vi "Measure Delay.vi"(0 "Oscilloscope in":refnum<class "Oscilloscope.lvclass">, 1 "From Slope Edge":T2, 5 "From Channel":T3, 7 "To Channel":T3, 9 "No. Reads":i32, 11 "error in (no error)":errorcluster, 12 "To Slope Edge":T2) -> (4 "Oscilloscope out":refnum<class "Oscilloscope.lvclass">, 6 "Statistics":T1, 15 "error out":errorcluster)   [LabVIEW 2018, in "Oscilloscope.lvlib" / "Oscilloscope.lvclass"]
doc: "This Override measure the signal time gap between From Channel's Slope Edge to To Channel's Slope Edge."
uses:
  Oscilloscope.lvclass
  Custom Controls/Analog Channels.ctl
  Custom Controls/Slope Edge.ctl
  Oscilloscope.lvlib
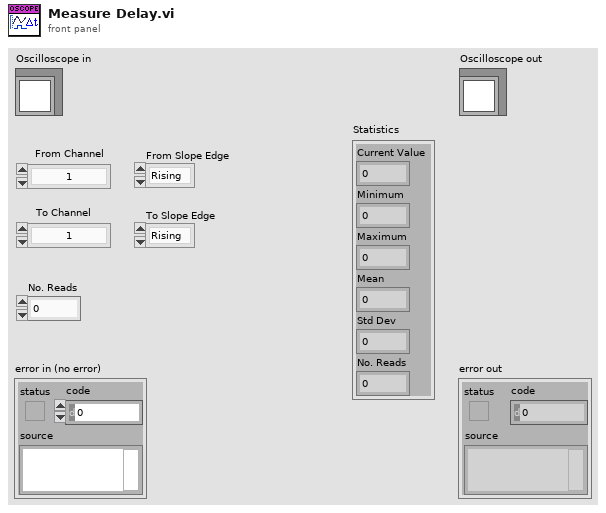
[diagram p1: front panel]
types:
  T1 = cluster{"Current Value":dbl, "Minimum":dbl, "Maximum":dbl, "Mean":dbl, "Std Dev":dbl, "No. Reads":dbl}
  T2 = typedef "Oscilloscope.lvlib/Slope Edge.ctl" = enum16{"Rising", "Falling"}
  T3 = typedef "Oscilloscope.lvlib/Analog Channels.ctl" = enum16{"1", "2", "3", "4", "5", "6", "7", "8", "9", "10", "11", "12", "13", "14", "15", "16"}
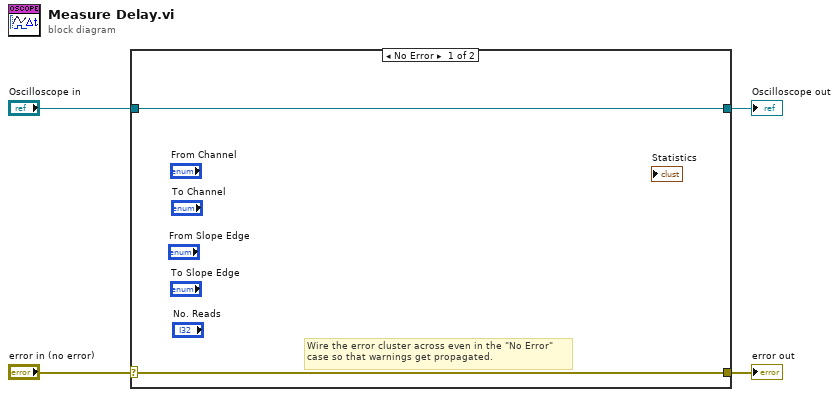
[diagram p0: block diagram]
diagram:
  n1 = case shown="No Error" "error in (no error)" {
    selector: "error in (no error)" -> [w5 w8]
    tunnel: [w5 w8] -> w3
    tunnel: [w6 w7] -> w1
    tunnel: "Oscilloscope in" -> [w6 w7]
    frame No Error {
      # "Wire the error cluster across even in the \"No Error\"\ncase so that warnings get propagated."
    }
    frame Error {
    }
  }
  "error out" <- w3
  "Oscilloscope out" <- w1
